vi "VITest1.vi"() -> ()   [LabVIEW 2012]
panel:
  out "Analog Input":i16[](array[numeric])
  in  "Click to stop program":bool
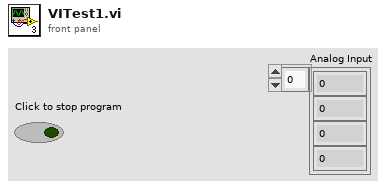
[diagram p1: front panel]
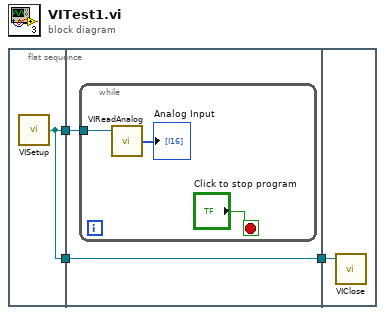
[diagram p0: block diagram]
diagram:
  n1 = flat-sequence {
    tunnel: [w4] -> w3
    tunnel: [w4] -> w2
    tunnel: w3 -> [w6]
    tunnel: w2 -> [w5]
    tunnel: [w5] -> w1
    tunnel: w1 -> [w10]
    frame #0 {
      n2 = call "VISetup.vi"() -> ("FPGA Interface Output"=w4:refnum<k20>)  [unwired: 1 in, 1 out]
    }
    frame #1 {
      n3 = while {
        tunnel: w6 -> [w9]
        stop <- "Click to stop program" stop-if-true
        n4 = call "VIReadAnalog.vi"("FPGA Interface Input"=w9) -> ("Analog Input"=→"Analog Input":i16[])  [unwired: 1 in]
      }
    }
    frame #2 {
      n5 = call "VIClose.vi"("FPGA Interface Input"=w10) -> ()  [unwired: 1 in, 1 out]
    }
  }
